vi "StringLengthValidation_SN.vi"(9 "NumbertoRestric":dbl, 10 "MessagetoDisplay":string, 11 "StringToValidate":string) -> (3 "StringAfterValidation":string)   [LabVIEW 2012]
panel:
  # "Function used to validate length of the string"
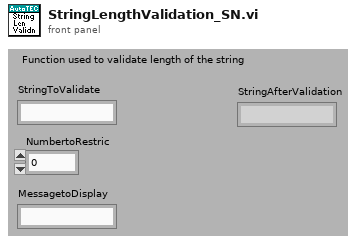
[diagram p1: front panel]
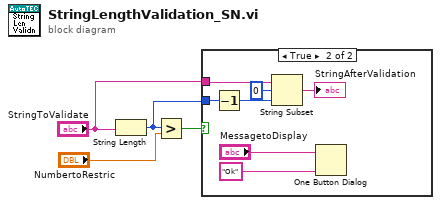
[diagram p0: block diagram]
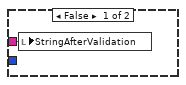
[diagram p2: hidden frame]
diagram:
  n1 = String Length(string="StringToValidate") -> (length=w3:i32)
  n2 = Greater?(x=w3, y="NumbertoRestric") -> (0:w4:bool)
  n3 = case shown="True" w4 {
    tunnel: "StringToValidate" -> [w5 w11]
    tunnel: w3 -> [_ w9]
    frame False {
      n4 = local write "StringAfterValidation"(w5) -> ()
    }
    frame True {
      n5 = Decrement(x=w9) -> (x-1=w8:i32)
      n6 = String Subset(string=w11, offset (0)=0, length (rest)=w8) -> (substring=→"StringAfterValidation":string)
      n7 = One Button Dialog(message="MessagetoDisplay", button name ("OK")="Ok") -> ()  [unwired: 1 out]
    }
  }
